vi "EventInfoTestCaseChange.vi"(8 "error in (no error)":errorcluster, 11 "TestCaseInfo":string[](array[string])=["project", "subfolder", "filename", "measurementnumber"]) -> (0 "error out":errorcluster, 3 "JSON Tree out (JSON Object)":variant)   [LabVIEW 2018]
uses:
  <vilib>/LVH/i3 JSON/JSON Generation/Create Value Files/Create Value - Object.vi
  <vilib>/LVH/i3 JSON/JSON Generation/Add Object Parameter Files/Add Object Parameter - String.vi
  <vilib>/LVH/i3 JSON/JSON Generation/Add Object Parameter Files/Add Object Parameter - Object.vi
  <vilib>/LVH/i3 JSON/i3-json.lvlib
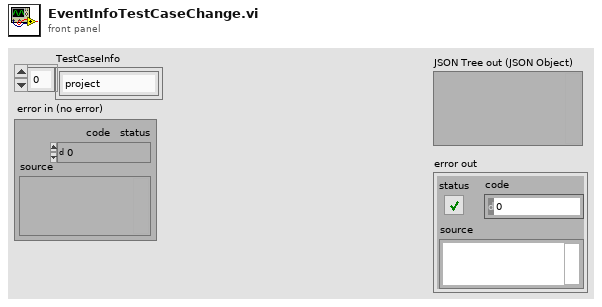
[diagram p1: front panel]
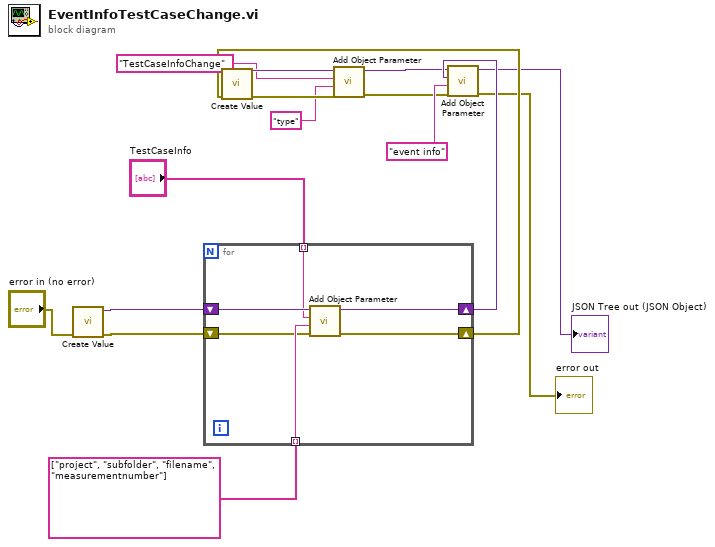
[diagram p0: block diagram]
diagram:
  n1 = call-poly <vilib>:"Create Value.vi"("error in (no error)"="error in (no error)") -> ("error out"=w13:errorcluster, "JSON Tree"=w15:variant)  [unwired: 9 in]
  n2 = for {
    tunnel: string[] ["project", "subfolder", "filename", "measurementnumber"] -> [w22] mode=indexing
    tunnel: "TestCaseInfo" -> [w20] mode=indexing
    shift-right: [w17] -> w9
    shift-left: w13 -> [w19]
    shift-right: [w18] -> w10
    shift-left: w15 -> [w21]
    n3 = call-poly <vilib>:"Add Object Parameter.vi"("error in (no error)"=w19, "Name"=w22, "String"=w20, "JSON Tree in (JSON Object)"=w21) -> ("error out"=w17:errorcluster, "JSON Tree out (JSON Object)"=w18:variant)  [unwired: 6 in]
  }
  n4 = call-poly <vilib>:"Create Value.vi"("error in (no error)"=w9) -> ("error out"=w8:errorcluster, "JSON Tree"=w5:variant)  [unwired: 9 in]
  n5 = call-poly <vilib>:"Add Object Parameter.vi"("error in (no error)"=w8, "Name"="type", "String"="TestCaseInfoChange", "JSON Tree in (JSON Object)"=w5) -> ("error out"=w7:errorcluster, "JSON Tree out (JSON Object)"=w6:variant)  [unwired: 6 in]
  n6 = call-poly <vilib>:"Add Object Parameter.vi"("error in (no error)"=w7, "Name"="event info", "JSON Object"=w10, "JSON Tree in (JSON Object)"=w6) -> ("error out"=→"error out":errorcluster, "JSON Tree out (JSON Object)"=→"JSON Tree out (JSON Object)":variant)  [unwired: 6 in]
